vi "Teleop Drivetrain Control.vi"(10 "Button Cluster":T1, 11 "Axes":T2) -> ()   [LabVIEW 2015]
uses:
  Common Code/Gamepads/Axes Cluster.ctl
  Common Code/Gamepads/Button Cluster.ctl
  Drivetrain Modes.ctl
  Robot Global Data.vi
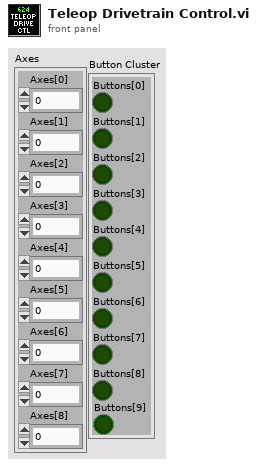
[diagram p1: front panel]
types:
  T1 = typedef "Button Cluster.ctl" = cluster{"Buttons[0]":bool, "Buttons[1]":bool, "Buttons[2]":bool, "Buttons[3]":bool, "Buttons[4]":bool, "Buttons[5]":bool, "Buttons[6]":bool, "Buttons[7]":bool, "Buttons[8]":bool, "Buttons[9]":bool}
  T2 = typedef "Axes Cluster.ctl" = cluster{"Axes[0]":dbl, "Axes[1]":dbl, "Axes[2]":dbl, "Axes[3]":dbl, "Axes[4]":dbl, "Axes[5]":dbl, "Axes[6]":dbl, "Axes[7]":dbl, "Axes[8]":dbl}
  T3 = typedef "Drivetrain Modes.ctl" = enum16{"Normal", "Cubic Profile", "Trapezoidal Profile", "Turn to Angle", "Distance Drive", "Data Acquisition"}
  T4 = typedef "Drivetrain Commands.ctl" = cluster{"Mode":T3, "Y Power":dbl, "Turn Power":dbl, "Distance":sgl}
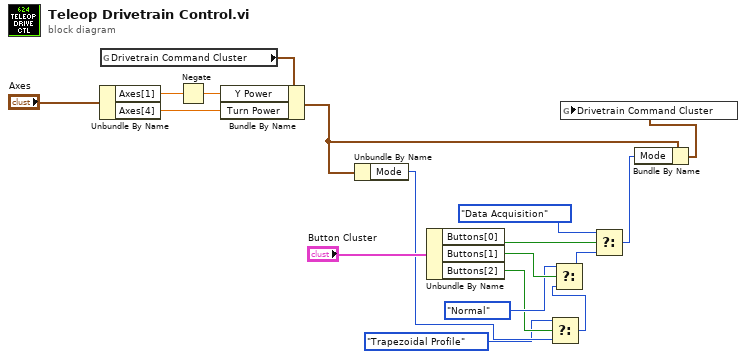
[diagram p0: block diagram]
diagram:
  n1 = Unbundle By Name("Axes") -> ("Axes[1]"=w6:dbl, "Axes[4]"=w16:dbl)
  n2 = global read "Robot Global Data.vi" "Drivetrain Command Cluster"() -> (w17:T4)
  n3 = Negate(x=w6) -> (-x=w5:dbl)
  n4 = Bundle By Name(cluster=w17, "Y Power"=w5, "Turn Power"=w16) -> (w9:T4)
  n5 = Unbundle By Name(w9) -> ("Mode"=w3:T3)
  n6 = Unbundle By Name("Button Cluster") -> ("Buttons[0]"=w14:bool, "Buttons[1]"=w12:bool, "Buttons[2]"=w4:bool)
  n7 = Select(t=Drivetrain_Modes."Trapezoidal Profile", s=w4, f=w3) -> (s? t:f=w1:T3)
  n8 = Select(t=Drivetrain_Modes."Normal", s=w12, f=w1) -> (s? t:f=w13:T3)
  n9 = Select(t=Drivetrain_Modes."Data Acquisition", s=w14, f=w13) -> (s? t:f=w8:T3)
  n10 = Bundle By Name(cluster=w9, "Mode"=w8) -> (w7:T4)
  n11 = global write "Robot Global Data.vi" "Drivetrain Command Cluster"(w7) -> ()
